vi "cut1.vi"(3 "start/duration format":u16(ring)=1 items=["Samples", "Relative Time"], 4 "data info template":refnum<vi>, 5 "input":waveform(dbl), 6 "open interval? (T)":bool, 7 "cut  end":dbl=0.001 format="%#.6e", 8 "cut start":dbl=0.01 format="%#.6e") -> (0 "Part of input":waveform(dbl), 1 "short cut data lables":string, 2 "cut data lables":string)   [LabVIEW 2014]
uses:
  <vilib>/Waveform/WDTOps.llb/WDT Get Waveform Subset DBL.vi
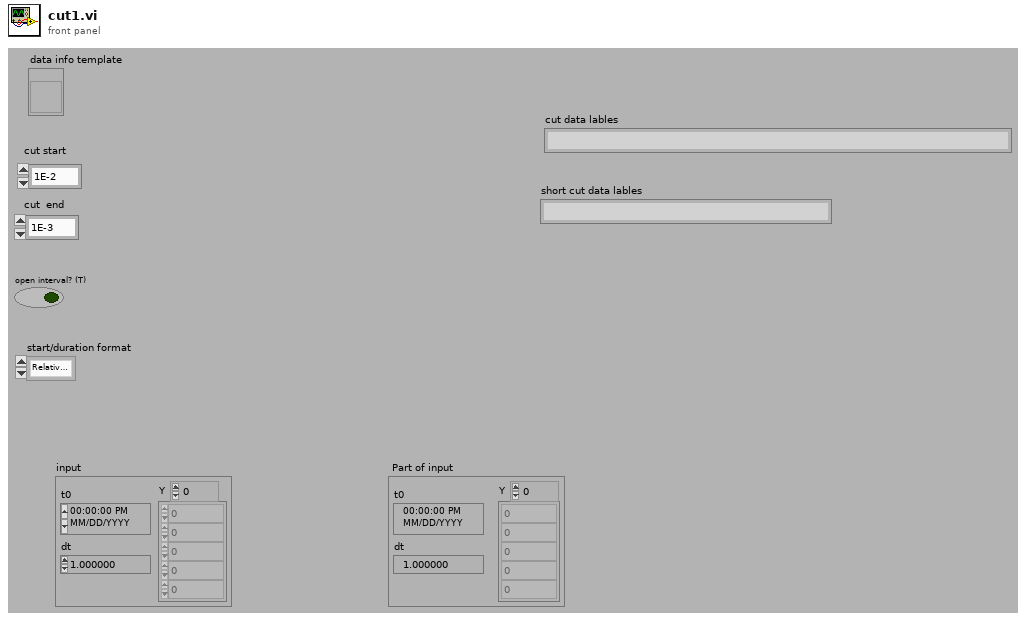
[diagram p1: front panel]
types:
  T1 = cluster{"data path":string, "ADCintercadr_s":dbl, "data info":cluster{"use or not *.info.txt?":i16, "probe name":string, "signal type":string, "Unit":string, "variable":string, "attenuation factor":dbl, "amplification factor":dbl, "extracoef#1":dbl, "extracoef#2":dbl, "U cascade, kV":string, "probe area, cm2":dbl, "plasma, a.m.u.":dbl}, "channel_name":string, "channels_in_file":i32, "LastModified":string}
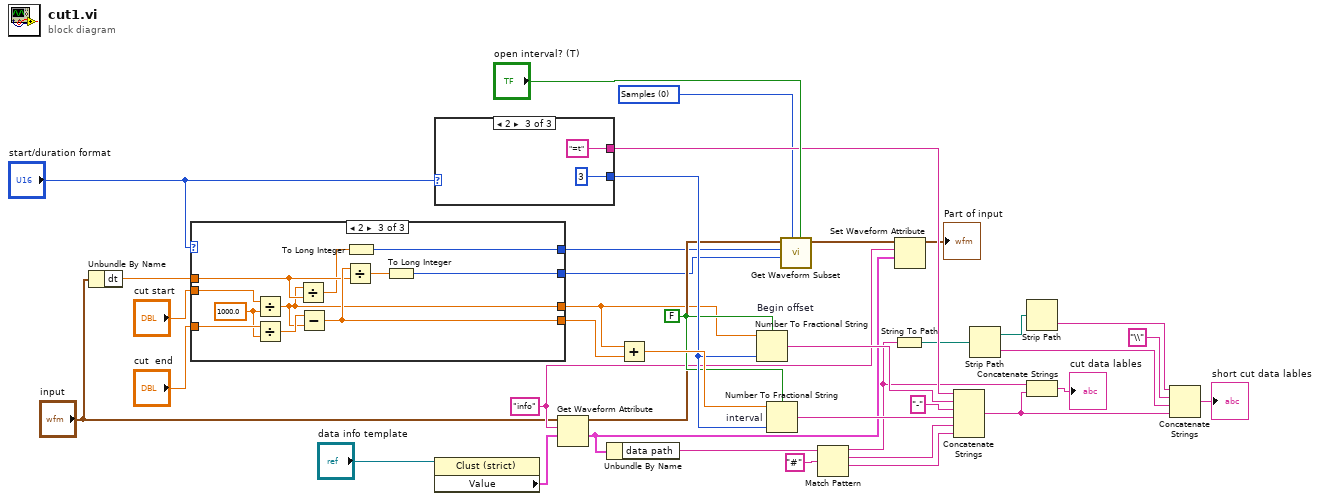
[diagram p0: block diagram]
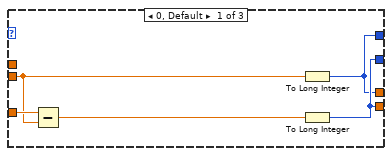
[diagram p2: hidden frame]
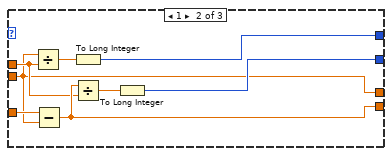
[diagram p3: hidden frame]
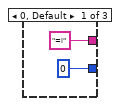
[diagram p4: hidden frame]
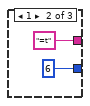
[diagram p5: hidden frame]
diagram:
  w7 = u16 0 items=["Samples", "Relative Time"] ("start/duration format")
  w18 = FALSE ("use system decimal point (T)")
  w16 = "info" ("name")
  n1 = Unbundle By Name("input") -> ("dt"=w5:dbl)
  n2 = case shown="2" "start/duration format" {
    tunnel: "cut  end" -> [w43 w51 w56]
    tunnel: [w41 w45 w57] -> w11
    tunnel: "cut start" -> [w40 w44 w55]
    tunnel: [w39 w47 w59] -> w9
    tunnel: w5 -> [_ w49 w61]
    tunnel: [w41 w50 w62] -> w4
    tunnel: [w39 w44 w52] -> w2
    frame 0, Default {
      n3 = Subtract(x=w43, y=w40) -> (x-y=w42:dbl)
      n4 = To Long Integer(number=w40) -> (32bit integer=w39:i32)
      n5 = To Long Integer(number=w42) -> (32bit integer=w41:i32)
    }
    frame 1 {
      n6 = Divide(x=w44, y=w49) -> (x/y=w48:dbl)
      n7 = Subtract(x=w51, y=w44) -> (x-y=w50:dbl)
      n8 = To Long Integer(number=w48) -> (32bit integer=w47:i32)
      n9 = Divide(x=w50, y=w49) -> (x/y=w46:dbl)
      n10 = To Long Integer(number=w46) -> (32bit integer=w45:i32)
    }
    frame 2 {
      w54 = 1000.0 ("y")
      n11 = Divide(x=w55, y=w54) -> (x/y=w52:dbl)
      n12 = Divide(x=w56, y=w54) -> (x/y=w53:dbl)
      n13 = Divide(x=w52, y=w61) -> (x/y=w60:dbl)
      n14 = Subtract(x=w53, y=w52) -> (x-y=w62:dbl)
      n15 = Divide(x=w62, y=w61) -> (x/y=w58:dbl)
      n16 = To Long Integer(number=w60) -> (32bit integer=w59:i32)
      n17 = To Long Integer(number=w58) -> (32bit integer=w57:i32)
    }
  }
  n18 = case shown="2" "start/duration format" {
    tunnel: [i16 0 ("precision (6)") i16 6 ("precision (6)") i16 3 ("precision (6)")] -> w34
    tunnel: ["=i" "=t" "=t"] -> w29
    frame 0, Default {
    }
    frame 1 {
    }
    frame 2 {
    }
  }
  n19 = property on="Property Node" class="Clust (strict)"(reference="data info template") -> ("Value"=w3:T1)  [unwired: 1 in, 2 out]
  n20 = Get Waveform Attribute(5:w3, 6:w16, 7:"input") -> (1:w14:T1, 3:w15:waveform(dbl))  [unwired: 1 in, 2 out]
  n21 = Unbundle By Name(w14) -> ("data path"=w17:string)
  n22 = Add(x=w2, y=w4) -> (x+y=w35:dbl)
  n23 = Number To Fractional String "Begin offset"(use system decimal point (T)=w18, number=w2, precision (6)=w34) -> (F-format string=w37:string)  [unwired: 1 out]
  n24 = Number To Fractional String "interval"(use system decimal point (T)=w18, number=w35, precision (6)=w34) -> (F-format string=w38:string)  [unwired: 1 out]
  n25 = call-poly <vilib>:"Get Waveform Subset.vi"("open interval? (T)"="open interval? (T)", "start/duration format"=w7, "duration"=w11, "start samples/time"=w9, "waveform in"=w15) -> ("waveform out"=w33:waveform(dbl))  [unwired: 1 in, 3 out]
  n26 = Match Pattern(string=w17, regular expression="#") -> (before substring=w27:string, match substring=w28:string, after substring=w20:string)  [unwired: 1 in, 1 out]
  n27 = String To Path(string=w27) -> (path=w26:path)
  n28 = Set Waveform Attribute(5:w14, 6:w16, 7:w33) -> (3:→"Part of input":waveform(dbl))  [unwired: 1 in, 2 out]
  n29 = Concatenate Strings(w29, w37, "-", w38, w28, w20) -> (w19:string)
  n30 = Strip Path(path=w26) -> (stripped path=w23:path, name=w25:string)
  n31 = Strip Path(path=w23) -> (name=w21:string)  [unwired: 1 out]
  n32 = Concatenate Strings(w27, w19) -> (→"cut data lables":string)
  n33 = Concatenate Strings(w21, "\\" ("string"), w25, w19) -> (→"short cut data lables":string)
